vi "Final-MurphyE-Main.vi"() -> ()   [LabVIEW 2019]
uses:
  <vilib>/Analysis/1siggen.llb/Ramp Pattern by Samples.vi
  <vilib>/Utility/file.llb/Write Delimited Spreadsheet (DBL).vi
  <vilib>/Analysis/NI_AALBase.lvlib
panel:
  out "Inductor Value":string
  out "Capacitor Value":string
  out "Resistor  Value":string
  out "Results":cluster{"Ramp Pattern":dbl[], dbl[]}[](graph)
  out "parameter array":dbl[](array[numeric])
  out "standard output array":dbl[][](array[numeric])
  out "standard output":string
  out "command\nstring":string
  out "appended array":dbl[][](array[numeric])
  out "Multi1? 2":refnum<visa-resource-name>
  out "LogSpacedFreqList":dbl[](array[numeric])
  out "Multi1?":refnum<visa-resource-name>
  out "FG missing?":bool
  out "FG FOUND":bool
  out "Multimeter(s) Missing":bool
  out "2 Multimeters Found 2":bool
  out "Multimeters COM Port Array":refnum<visa-resource-name>[](array[refnum])
  # "Eddie Murphy's RLC Circuit Solver"
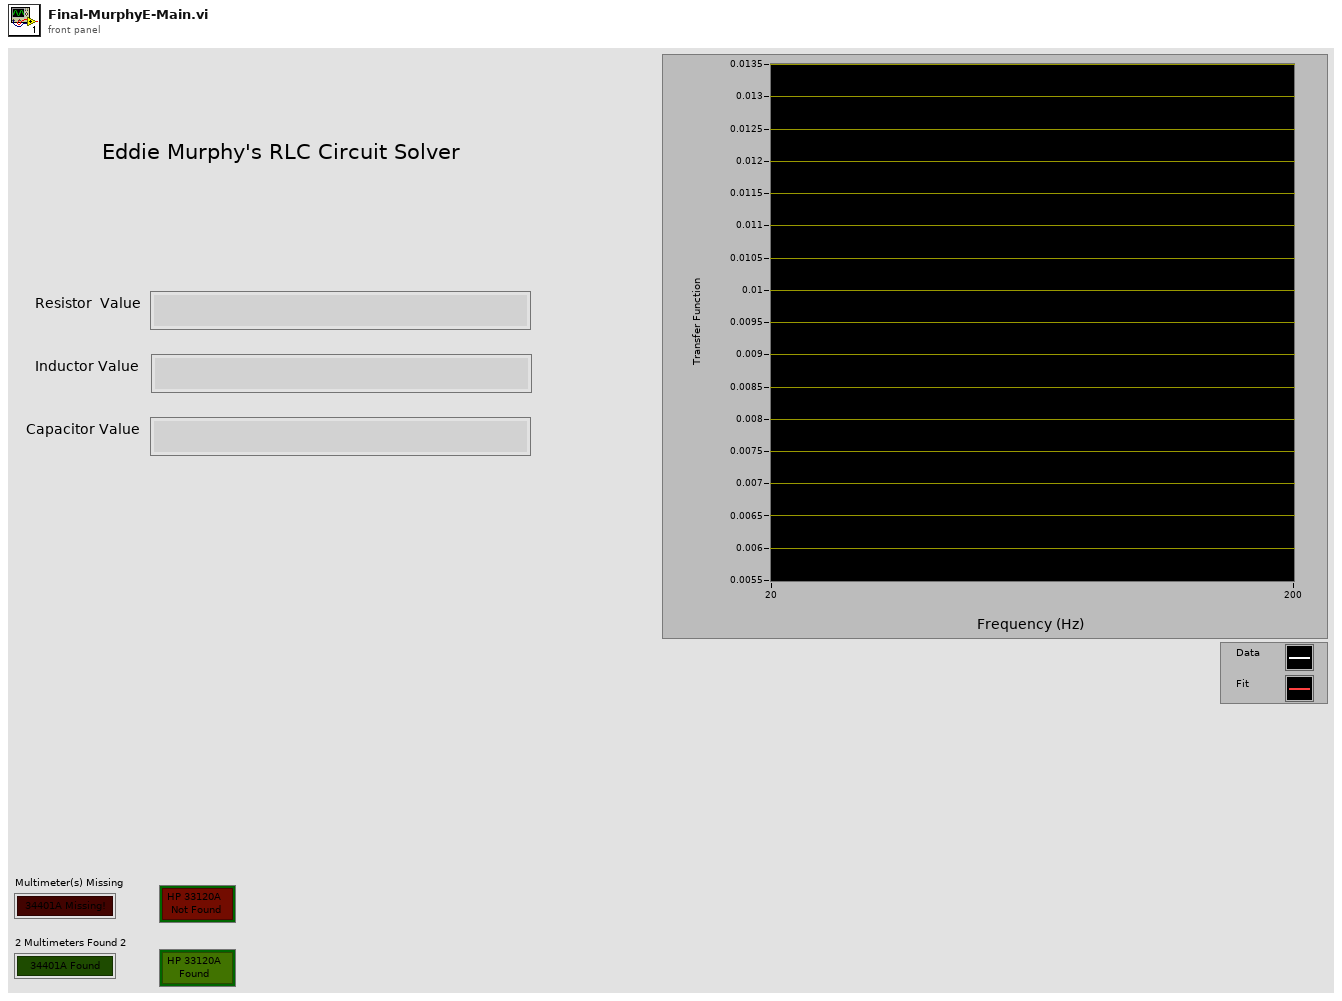
[diagram p1: front panel]
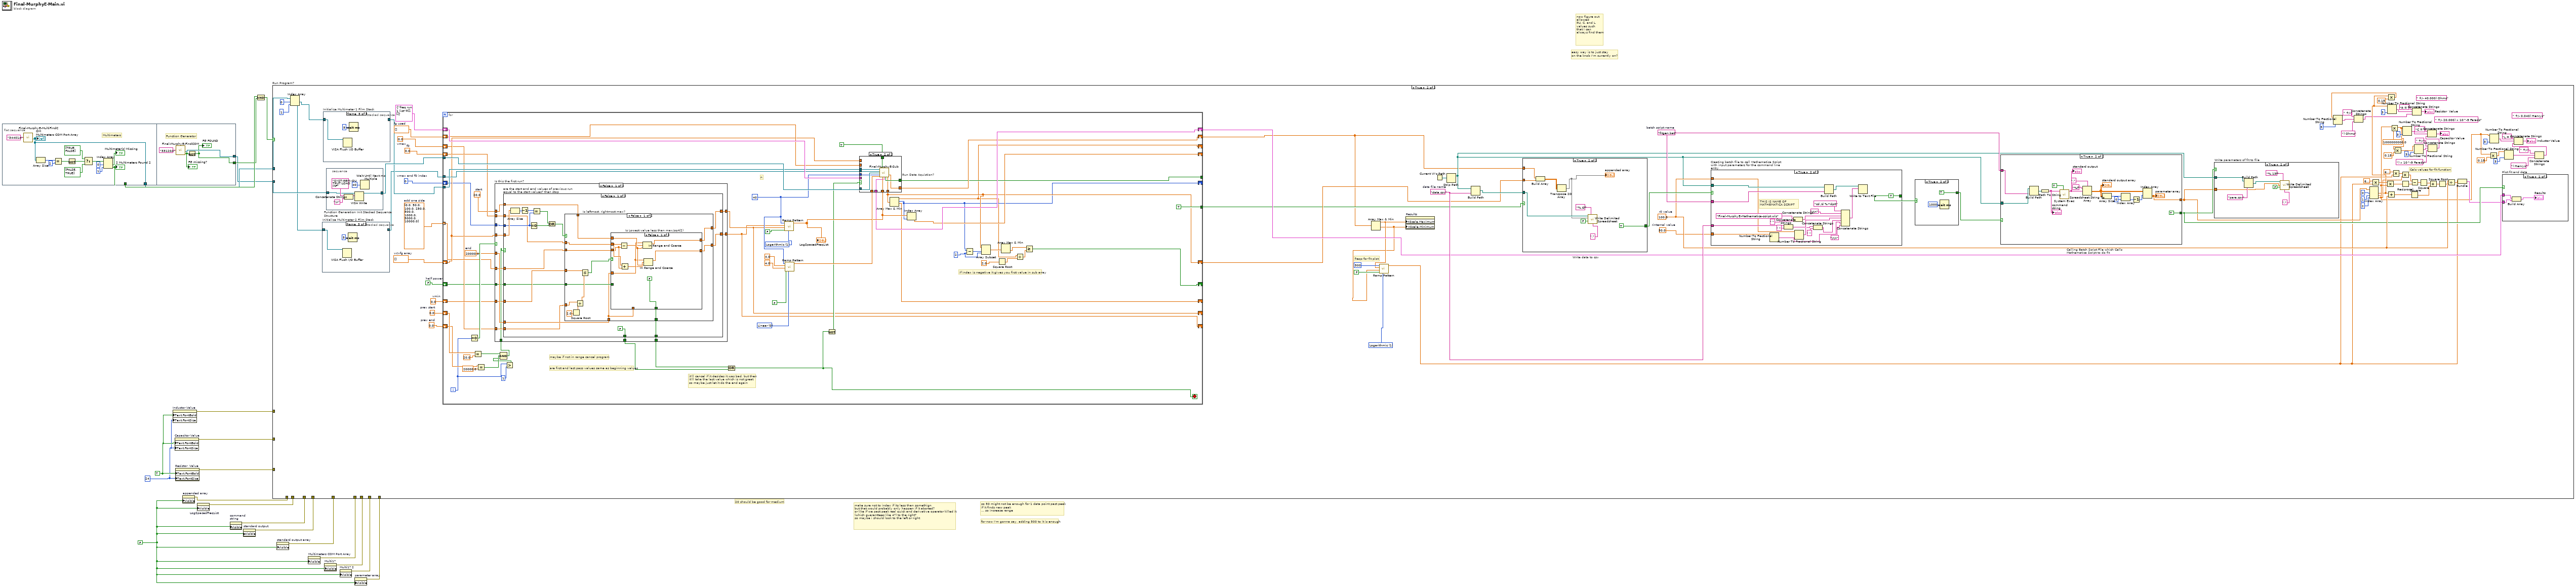
[diagram p0: block diagram]
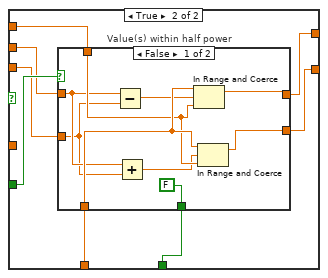
[diagram p3: hidden frame]
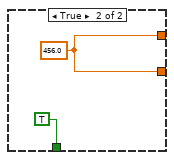
[diagram p4: hidden frame]
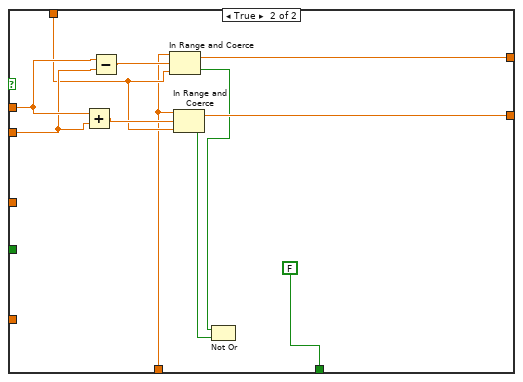
[diagram p5: hidden frame]
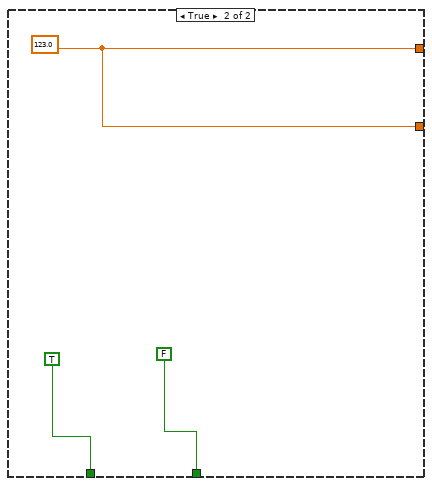
[diagram p6: hidden frame]
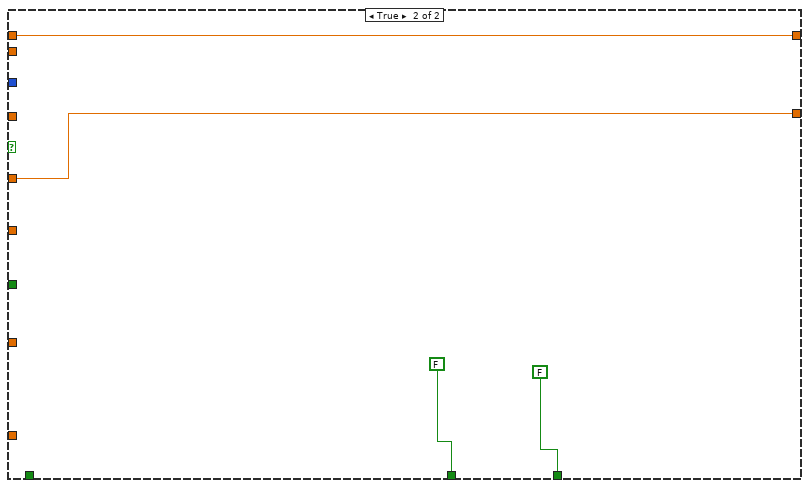
[diagram p7: hidden frame]
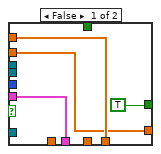
[diagram p8: hidden frame]
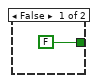
[diagram p11: hidden frame]
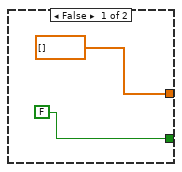
[diagram p12: hidden frame]
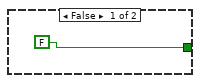
[diagram p13: hidden frame]
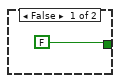
[diagram p14: hidden frame]
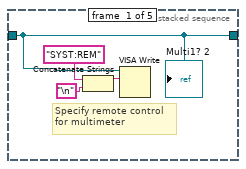
[diagram p15: hidden frame]
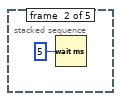
[diagram p16: hidden frame]
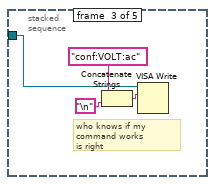
[diagram p17: hidden frame]
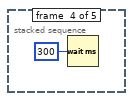
[diagram p18: hidden frame]
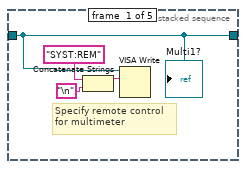
[diagram p19: hidden frame]
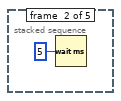
[diagram p20: hidden frame]
diagram:
  w3 = u32 24 ("Text.Font:Size")
  w4 = TRUE
  w7 = FALSE
  # "for now I'm gonna say, adding 500 to it is enough"
  # "so 50 might not be enough for 1 data point past peak\nif it finds new peak \n... so increase range"
  # "make sure not to index if its less than somethign\nbut that would probably only happen if it aborted?\nor like if we past peak real quick and derivative operator killed it (which guaranttees like 4?) to the right?\nso maybe i should look to the left or right"
  # "20 should be good for medium"
  # "easy way is to just stay \non the knob I'm currently on?"
  # "now figure out\nallowed\nRU, C, and L\nvalues such \nthat I can \nalways find them"
  n1 = flat-sequence {
    tunnel: [w22] -> w20
    tunnel: [w21] -> w18
    tunnel: [w36] -> w16
    tunnel: [w34] -> w19
    frame #0 {
      # "Multimeters"
      n2 = call "Final-MurphyE-MultiFindCOM.vi"("Name of Desired\nInstrument"="34401A" ("y")) -> ("Desired COM Port Array"=w21:refnum<visa-resource-name>[])  [unwired: 3 out]
      "Multimeters COM Port Array" <- w21
      n3 = Array Size(array=w21) -> (size(s)=w26:i32)
      n4 = Equal?(x=w26, y=2) -> (x = y?=w24:bool)
      n5 = Not(x=w24) -> (.not. x?=w23:bool)
      n6 = Select(t=bool[] [TRUE, FALSE], s=w23, f=bool[] [FALSE, TRUE]) -> (s? t:f=w30:bool[])
      n7 = Index Array(array=w30, index #1=0 ("index"), index #2=1) -> (element #1=→"Multimeter(s) Missing":bool, element #2=w22:bool)
      "2 Multimeters Found 2" <- w22
    }
    frame #1 {
      # "Function Generator"
      n8 = call "Final-MurphyE-FindCOM.vi"("Name of Desired\nInstrument"="33120A" ("y")) -> ("Desired \nCOM Port"=w36:refnum<visa-resource-name>, "Instrument\nNot Found"=w35:bool)  [unwired: 2 out]
      "FG missing?" <- w35
      n9 = Not(x=w35) -> (.not. x?=w34:bool)
      "FG FOUND" <- w34
    }
  }
  n10 = property on="Inductor Value" class="Str"("Text.FontBold"=w4, "Text.FontSize"=w3) -> (error out=w2:errorcluster)  [unwired: 2 in, 1 out]
  n11 = property on="Capacitor Value" class="Str"("Text.FontBold"=w4, "Text.FontSize"=w3) -> (error out=w1:errorcluster)  [unwired: 2 in, 1 out]
  n12 = property on="Resistor  Value" class="Str"("Text.FontBold"=w4, "Text.FontSize"=w3) -> (error out=w5:errorcluster)  [unwired: 2 in, 1 out]
  n13 = property on="appended array" class="Arr (strict)"("Visible"=w7) -> (error out=w14:errorcluster)  [unwired: 2 in, 1 out]
  n14 = property on="LogSpacedFreqList" class="Arr (strict)"("Visible"=w7) -> (error out=w15:errorcluster)  [unwired: 2 in, 1 out]
  n15 = property on="command\nstring" class="Str"("Visible"=w7) -> (error out=w13:errorcluster)  [unwired: 2 in, 1 out]
  n16 = property on="standard output" class="Str"("Visible"=w7) -> (error out=w12:errorcluster)  [unwired: 2 in, 1 out]
  n17 = Compound Arithmetic op=AND(w20, w19) -> (w17:bool)
  n18 = property on="standard output array" class="Arr (strict)"("Visible"=w7) -> (error out=w11:errorcluster)  [unwired: 2 in, 1 out]
  n19 = property on="Multimeters COM Port Array" class="Arr (strict)"("Visible"=w7) -> (error out=w8:errorcluster)  [unwired: 2 in, 1 out]
  n20 = property on="Multi1?" class="VISAName"("Visible"=w7) -> (error out=w10:errorcluster)  [unwired: 2 in, 1 out]
  n21 = property on="Multi1? 2" class="VISAName"("Visible"=w7) -> (error out=w9:errorcluster)  [unwired: 2 in, 1 out]
  n22 = property on="parameter array" class="Arr (strict)"("Visible"=w7) -> (error out=w6:errorcluster)  [unwired: 2 in, 1 out]
  n23 = case "Run Program?" shown="True" w17 {
    tunnel: w18 -> [_ w133]
    tunnel: w16 -> [_ w132]
    tunnel: w15 -> [_ _]
    tunnel: w14 -> [_ _]
    tunnel: w13 -> [_ _]
    tunnel: w12 -> [_ _]
    tunnel: w11 -> [_ _]
    tunnel: w10 -> [_ _]
    tunnel: w9 -> [_ _]
    tunnel: w8 -> [_ _]
    tunnel: w6 -> [_ _]
    tunnel: w5 -> [_ _]
    tunnel: w2 -> [_ _]
    tunnel: w1 -> [_ _]
    frame False {
    }
    frame True {
      w62 = FALSE  # half power
      w63 = 0.0  # prev end
      w64 = 0.0  # prev start
      w65 = 0.0  # vmin
      w66 = dbl[] [0.0, 50.0, 100.0, 250.0, 500.0, 1000.0, 5000.0, 10000.0]  # add one side
      w73 = u16 1 items=["Linear", "Logarithmic"] ("type")
      w80 = dbl[] []  # fg used
      w82 = 0.0  # vmax
      w83 = 0.0  # f0
      w84 = 0  # vmax and f0 index
      w85 = dbl[] []  # vr/vfg array
      w86 = 50.0  # rinternal value
      (unwired) " +/- 0.040) Henrys" ("string")
      (unwired) " +/- 20.000) x 10^-9 Farads" ("string")
      (unwired) " +/- 40.000) Ohms" ("string")
      w118 = 100.0  # r0 value
      w126 = "fitgen.bat"  # batch script name
      w123 = "data.csv"  # data file name
      # "freqs for fit plot"
      # "Calc values for fit function"
      n24 = Index Array(array=w133, index #1=0 ("index"), index #2=1 ("index")) -> (element #1=w131:refnum<visa-resource-name>, element #2=w130:refnum<visa-resource-name>)
      n25 = stacked-sequence "Initialize Multimeter 2 Film Stack" {
        tunnel: w130 -> [w362 _ w367 _ w372]
        tunnel: [w362 _ _ _ _] -> w75
        frame #0 {
          # "Specify remote control\nfor multimeter"
          n26 = Concatenate Strings("SYST:REM", "\n") -> (w365:string)
          n27 = VISA Write(VISA resource name=w362, write buffer=w365) -> ()  [unwired: 1 in, 3 out]
          "Multi1? 2" <- w362
        }
        frame #1 {
          n28 = Wait (ms)(milliseconds to wait=u32 5 ("millisecond multiple")) -> ()  [unwired: 1 out]
        }
        frame #2 {
          # "who knows if my command works\nis right"
          n29 = Concatenate Strings("conf:VOLT:ac", "\n") -> (w368:string)
          n30 = VISA Write(VISA resource name=w367, write buffer=w368) -> ()  [unwired: 1 in, 3 out]
        }
        frame #3 {
          n31 = Wait (ms)(milliseconds to wait=u32 300 ("millisecond multiple")) -> ()  [unwired: 1 out]
        }
        frame #4 {
          n32 = VISA Flush I/O Buffer(VISA resource name=w372) -> ()  [unwired: 2 in, 2 out]
          n33 = Wait (ms)(milliseconds to wait=u32 5 ("millisecond multiple")) -> ()  [unwired: 1 out]
        }
      }
      n34 = stacked-sequence "Initialize Multimeter 1 Film Stack" {
        tunnel: w131 -> [w380 _ w385 _ w390]
        tunnel: [w380 _ _ _ _] -> w76
        frame #0 {
          # "Specify remote control\nfor multimeter"
          n35 = Concatenate Strings("SYST:REM", "\n") -> (w383:string)
          n36 = VISA Write(VISA resource name=w380, write buffer=w383) -> ()  [unwired: 1 in, 3 out]
          "Multi1?" <- w380
        }
        frame #1 {
          n37 = Wait (ms)(milliseconds to wait=u32 5 ("millisecond multiple")) -> ()  [unwired: 1 out]
        }
        frame #2 {
          # "who knows if my command works\nis right"
          n38 = Concatenate Strings("conf:VOLT:ac", "\n") -> (w386:string)
          n39 = VISA Write(VISA resource name=w385, write buffer=w386) -> ()  [unwired: 1 in, 3 out]
        }
        frame #3 {
          n40 = Wait (ms)(milliseconds to wait=u32 300 ("millisecond multiple")) -> ()  [unwired: 1 out]
        }
        frame #4 {
          n41 = VISA Flush I/O Buffer(VISA resource name=w390) -> ()  [unwired: 2 in, 2 out]
          n42 = Wait (ms)(milliseconds to wait=u32 5 ("millisecond multiple")) -> ()  [unwired: 1 out]
        }
      }
      n43 = stacked-sequence "Function Generation Init Stacked Sequence Structure" {
        tunnel: w132 -> [w376]
        tunnel: [w374] -> w77
        frame #0 {
          n44 = Concatenate Strings("SYST:REM;:OUTPUT:LOAD INF", "\n") -> (w378:string)
          n45 = VISA Write(VISA resource name=w376, write buffer=w378) -> (VISA resource name out=w374:refnum<visa-resource-name>)  [unwired: 1 in, 2 out]
          n46 = Wait Until Next ms Multiple(millisecond multiple=u32 40) -> ()  [unwired: 1 out]
        }
      }
      n47 = for {
        tunnel: [w181] -> _
        shift-right: [w150] -> w78
        shift-left: w85 -> [w172]
        shift-right: [w148] -> _
        shift-left: w84 -> [w171]
        shift-right: [w175] -> _
        shift-left: w83 -> [w173]
        shift-right: [w141] -> _
        shift-left: w82 -> [w164]
        shift-right: [w185] -> w79
        shift-left: cluster{"freq run 1 list":dbl[], dbl[]} {"freq run 1 list"=[], []} ("vr/vfg rms Cluster for graph") -> [w184]
        shift-right: [w183] -> w68
        shift-left: w80 -> [w182]
        tunnel: w77 -> [w179]
        tunnel: w76 -> [w178]
        tunnel: w75 -> [w177]
        tunnel: [TRUE] -> w74
        tunnel: w66 -> [w168] mode=indexing
        shift-right: [w167] -> _
        shift-left: w65 -> [w166]
        shift-right: [w160] -> _
        shift-left: w64 -> [w158]
        shift-right: [w159] -> _
        shift-left: w63 -> [w156]
        shift-right: [w140] -> _
        shift-left: w62 -> [w139]
        i -> [w138]
        stop <- w161 stop-if-true
        w147 = 2
        w165 = 40
        w169 = 20000.0  # end
        w170 = 20.0  # start
        w187 = u16 1 items=["Linear", "Logarithmic"] ("type")
        w192 = u16 0 items=["Linear", "Logarithmic"] ("type")
        # "if index is negative it gives you first value in sub array"
        # "are first and last pass values same as beginning values"
        # "it'll cancel if it desides it was bad, but then \nit'll take the last value which is not great \nso maybe just let it do the end again"
        # "maybe if not in range cancel program"
        # "n"
        n48 = Equal To 0?(x=w138) -> (x = 0?=w174:bool)
        n49 = Equal?(x=w158, y=20.0) -> (x = y?=w154:bool)
        n50 = Equal?(x=w156, y=20000.0) -> (x = y?=w153:bool)
        n51 = Greater?(x=w138, y=1) -> (0:w136:bool)
        n52 = Compound Arithmetic op=AND(w154, w153, w136) -> (w152:bool)
        n53 = case "Is this the first run?" shown="False" w174 {
          tunnel: [w201 w285] -> w160
          tunnel: [w200 w284] -> w159
          tunnel: w173 -> [w205 _]
          tunnel: w172 -> [w207 _]
          tunnel: w171 -> [w206 _]
          tunnel: w170 -> [w204 w285]
          tunnel: w169 -> [w203 w284]
          tunnel: w168 -> [w202 _]
          tunnel: w166 -> [w199 _]
          tunnel: w164 -> [w198 _]
          tunnel: [w197 FALSE] -> w163
          tunnel: w152 -> [w196 _]
          tunnel: [w195 FALSE] -> w151
          tunnel: w139 -> [w194 _]
          frame False {
            n54 = case "are the start and end values of previous run equal to the start values? then stop" shown="False" w196 {
              tunnel: w207 -> [w224 _]
              tunnel: w206 -> [w221 _]
              tunnel: w205 -> [w218 _]
              tunnel: w204 -> [w217 _]
              tunnel: w203 -> [w216 _]
              tunnel: w202 -> [w215 _]
              tunnel: [w214 w281] -> w201
              tunnel: [w213 w281] -> w200
              tunnel: w199 -> [w212 _]
              tunnel: w198 -> [w211 _]
              tunnel: [w210 FALSE] -> w197
              tunnel: [FALSE TRUE] -> w195
              tunnel: w194 -> [w208 _]
              frame False {
                n55 = Array Size(array=w224) -> (size(s)=w223:i32)
                n56 = Decrement(x=w223) -> (x-1=w222:i32)
                n57 = Equal To 0?(x=w221) -> (x = 0?=w225:bool)
                n58 = Equal?(x=w222, y=w221) -> (x = y?=w220:bool)
                n59 = Or(x=w220, y=w225) -> (x .or. y?=w219:bool)
                n60 = case "Is leftmost, rightmost max?" shown="False" w219 {
                  tunnel: w218 -> [w229 w276]
                  tunnel: w217 -> [w230 w271]
                  tunnel: w216 -> [w226 w270]
                  tunnel: [w232 w278] -> w214
                  tunnel: [w231 w277] -> w213
                  tunnel: w215 -> [w228 w275]
                  tunnel: w212 -> [w239 _]
                  tunnel: w211 -> [w237 _]
                  tunnel: [w233 FALSE] -> w210
                  tunnel: w208 -> [w227 _]
                  frame False {
                    n61 = Square Root(x=2.0) -> (sqrt(x)=w235:dbl)
                    n62 = Divide(x=w237, y=w235) -> (x/y=w236:dbl)
                    n63 = Less Or Equal?(x=w239, y=w236) -> (x <= y?=w238:bool)
                    n64 = case "Is Lowest value less than max/sqrt(2)" shown="False" w238 {
                      tunnel: [FALSE w255] -> w233
                      tunnel: [w247 w254] -> w232
                      tunnel: [w246 w253] -> w231
                      tunnel: w226 -> [w244 _]
                      tunnel: w230 -> [w245 w251]
                      tunnel: w229 -> [w241 w250]
                      tunnel: w228 -> [w240 w249]
                      tunnel: w227 -> [_ w256]
                      tunnel: w226 -> [_ w252]
                      frame False {
                        n65 = Subtract(x=w241, y=w240) -> (x-y=w243:dbl)
                        n66 = Add(x=w241, y=w240) -> (x+y=w242:dbl)
                        n67 = In Range and Coerce(upper limit=w244, x=w243, lower limit=w245) -> (coerced(x)=w247:dbl)  [unwired: 1 out]
                        n68 = In Range and Coerce(upper limit=w244, x=w242, lower limit=w245) -> (coerced(x)=w246:dbl)  [unwired: 1 out]
                      }
                      frame True {
                        n69 = case "Value(s) within half power" shown="False" w256 {
                          tunnel: [FALSE TRUE] -> w255
                          tunnel: [w259 w266] -> w254
                          tunnel: [w260 w266] -> w253
                          tunnel: w252 -> [w264 _]
                          tunnel: w251 -> [w263 _]
                          tunnel: w250 -> [w258 _]
                          tunnel: w249 -> [w257 _]
                          frame False {
                            n70 = Subtract(x=w258, y=w257) -> (x-y=w262:dbl)
                            n71 = Add(x=w258, y=w257) -> (x+y=w261:dbl)
                            n72 = In Range and Coerce(upper limit=w264, x=w262, lower limit=w263) -> (coerced(x)=w259:dbl)  [unwired: 1 out]
                            n73 = In Range and Coerce(upper limit=w264, x=w261, lower limit=w263) -> (coerced(x)=w260:dbl)  [unwired: 1 out]
                          }
                          frame True {
                            w266 = 456.0
                          }
                        }
                      }
                    }
                  }
                  frame True {
                    n74 = Add(x=w276, y=w275) -> (x+y=w274:dbl)
                    n75 = Subtract(x=w276, y=w275) -> (x-y=w273:dbl)
                    n76 = In Range and Coerce(upper limit=w270, x=w273, lower limit=w271) -> (coerced(x)=w278:dbl, In Range?=w268:bool)
                    n77 = In Range and Coerce(upper limit=w270, x=w274, lower limit=w271) -> (coerced(x)=w277:dbl, In Range?=w269:bool)
                    n78 = Not Or(1:w269, 2:w268) -> ()  [unwired: 1 out]
                  }
                }
              }
              frame True {
                w281 = 123.0
              }
            }
          }
          frame True {
          }
        }
        n79 = Compound Arithmetic op=OR(w163, w151) -> (w161:bool)
        n80 = call-poly <vilib>:"Ramp Pattern.vi"("type"=w187, "exclude end?"=FALSE, "start"=w160, "end"=w159, "samples"=w165) -> ("Ramp Pattern"=w186:dbl[])  [unwired: 5 in, 1 out]
        "LogSpacedFreqList" <- w186
        n81 = call-poly <vilib>:"Ramp Pattern.vi"("type"=w192, "exclude end?"=FALSE, "start"=4.0, "end"=4.0, "samples"=w165) -> ("Ramp Pattern"=w188:dbl[])  [unwired: 5 in, 1 out]
        n82 = Not(x=w161) -> (.not. x?=w162:bool)
        n83 = case "Run Data Aquistion?" shown="True" w162 {
          tunnel: w178 -> [_ w300]
          tunnel: w177 -> [_ w299]
          tunnel: w179 -> [_ w298]
          tunnel: w188 -> [_ w297]
          tunnel: TRUE ("Measure? 2 Init Value") -> [_ w296]
          tunnel: [TRUE w295] -> w181
          tunnel: w165 -> [_ w294]
          tunnel: w186 -> [_ w293]
          tunnel: [w289 w292] -> w150
          tunnel: w172 -> [w289 _]
          tunnel: [w287 w291] -> w185
          tunnel: w184 -> [w287 _]
          tunnel: [w286 w290] -> w183
          tunnel: w182 -> [w286 _]
          frame False {
          }
          frame True {
            n84 = call "Final-MurphyE-Sub.vi"("multimeter 1 in"=w300, "Measure? 2 Init Value"=w296, "multimeter 2 in"=w299, "function gen in"=w298, "n"=w294, "vp-pk to pk array of values"=w297, "freq array input"=w293) -> ("freq array output (used)"=w290:dbl[], "vr/vfg rms Cluster for graph"=w291:cluster{"freq run 1 list":dbl[], dbl[]}, "Run 2 True Condition Measure Button"=w295:bool, "vr/vfg array"=w292:dbl[])  [unwired: 1 in, 4 out]
          }
        }
        n85 = Array Max & Min(array=w150) -> (max value=w141:dbl, max index (indices)=w148:i32, min value=w167:dbl)  [unwired: 1 out]
        n86 = Index Array(array=w186, index=w148) -> (element=w175:dbl)
        n87 = Subtract(x=w148, y=w147) -> (x-y=w149:i32)
        n88 = Array Subset(array=w150, index=w149, length=w147) -> (w146:dbl[])
        n89 = Square Root(x=2.0) -> (sqrt(x)=w143:dbl)
        n90 = Array Max & Min(array=w146) -> (min value=w145:dbl)  [unwired: 3 out]
        n91 = Divide(x=w141, y=w143) -> (x/y=w144:dbl)
        n92 = Greater Or Equal?(x=w145, y=w144) -> (x >= y?=w140:bool)
      }
      n93 = Array Max & Min(array=w68) -> (max value=w70:dbl, min value=w69:dbl)  [unwired: 2 out]
      n94 = call-poly <vilib>:"Ramp Pattern.vi"("type"=w73, "exclude end?"=FALSE, "start"=w69, "end"=w70, "samples"=500) -> ("Ramp Pattern"=w67:dbl[])  [unwired: 5 in, 1 out]
      n95 = property on="Results" class="XYGraph (strict)"("XScale.Maximum"=w70, "XScale.Minimum"=w69) -> ()  [unwired: 2 in, 2 out]
      n96 = Current VI's Path() -> (path=w128:path)
      n97 = Strip Path(path=w128) -> (stripped path=w104:path)  [unwired: 1 out]
      n98 = Build Path(base path=w104, name or relative path=w123) -> (appended path=w127:path)
      n99 = case "Write data to csv" shown="True" w74 {
        tunnel: w68 -> [_ w361]
        tunnel: w78 -> [_ w360]
        tunnel: [FALSE TRUE] -> w129
        tunnel: w127 -> [_ w356]
        frame False {
        }
        frame True {
          n100 = Build Array(w361, w360) -> (w355:dbl[][])
          n101 = Transpose 2D Array(2D array=w355) -> (transposed array=w354:dbl[][])
          "appended array" <- w354
          n102 = call-poly <vilib>:"Write Delimited Spreadsheet.vi"("file path (dialog if empty)"=w356, "format (%.3f)"="%.6f", "2D data"=w354, "append to file? (new file:F)"=FALSE, "delimiter (\\t)"="," ("delimiter (\\t)")) -> ()  [unwired: 9 in, 2 out]
        }
      }
      n103 = case "Creating batch file to call Mathematica Script with input parameters for the command line entry" shown="True" w129 {
        tunnel: [FALSE TRUE] -> w125
        tunnel: w104 -> [_ w346]
        tunnel: w126 -> [_ w345]
        tunnel: w123 -> [_ w344]
        tunnel: w118 -> [_ w341]
        tunnel: w86 -> [_ w332]
        frame False {
        }
        frame True {
          # "THIS IS NAME OF \nMATHEMATICA SCRIPT"
          n104 = Number To Fractional String(number=w332) -> (F-format string=w339:string)  [unwired: 3 in]
          n105 = Concatenate Strings(w344, " " ("string")) -> (w342:string)
          n106 = Concatenate Strings("Final-MurphyE-Mathematica-script.wls" ("string"), " " ("string")) -> (w337:string)
          n107 = Number To Fractional String(number=w341) -> (F-format string=w335:string)  [unwired: 3 in]
          n108 = Concatenate Strings(w335, " " ("string")) -> (w334:string)
          n109 = Build Path(base path=w346, name or relative path=w345) -> (appended path=w350:path)
          n110 = Concatenate Strings("cd /d %~dp0" ("string"), "\r\n", w337, w342, w334, w339, "\r\n") -> (w349:string)
          n111 = Write to Text File(file (use dialog)=w350, text=w349) -> ()  [unwired: 2 in, 3 out]
        }
      }
      n112 = case shown="True" w125 {
        tunnel: [FALSE TRUE] -> w124
        frame False {
        }
        frame True {
          n113 = Wait (ms)(milliseconds to wait=u32 1000) -> ()  [unwired: 1 out]
        }
      }
      n114 = case "Calling Batch Script File which Calls Mathematica Script to do fit" shown="True" w124 {
        tunnel: w104 -> [_ w319]
        tunnel: w126 -> [_ w318]
        tunnel: [FALSE TRUE] -> w103
        tunnel: [dbl[] [] w316] -> w101
        frame False {
        }
        frame True {
          n115 = Build Path(base path=w319, name or relative path=w318) -> (appended path=w330:path)
          n116 = Path To String(path=w330) -> (string=w328:string)
          "command\nstring" <- w328
          n117 = call <vilib>:"System Exec.vi"("wait until completion? (T)"=TRUE, "command line"=w328) -> ("standard output"=w327:string)  [unwired: 6 in, 3 out]
          "standard output" <- w327
          n118 = Spreadsheet String To Array(delimiter (Tab)=",", format string="%f", spreadsheet string=w327) -> (array=w321:dbl[][])  [unwired: 1 in]
          "standard output array" <- w321
          n119 = Array Size(array=w321) -> (size(s)=w324:i32[])
          n120 = Index Array(array=w324, index=0) -> (element=w322:i32)
          n121 = Decrement(x=w322) -> (x-1=w320:i32)
          n122 = Index Array(array=w321, index (row)=w320) -> (element=w316:dbl[])  [unwired: 1 in]
          "parameter array" <- w316
        }
      }
      n123 = case "Write parameters of fit to file" shown="True" w103 {
        tunnel: w104 -> [_ w303]
        tunnel: w101 -> [_ w302]
        frame False {
        }
        frame True {
          n124 = Build Path(base path=w303, name or relative path="para.csv") -> (appended path=w305:path)
          n125 = call-poly <vilib>:"Write Delimited Spreadsheet.vi"("file path (dialog if empty)"=w305, "format (%.3f)"="%.13f", "1D data"=w302, "append to file? (new file:F)"=FALSE, "delimiter (\\t)"="," ("delimiter (\\t)")) -> ()  [unwired: 9 in, 2 out]
        }
      }
      n126 = Index Array(array=w101, index #1=0 ("index"), index #2=1 ("index"), index #3=2 ("index")) -> (element #1=w61:dbl, element #2=w94:dbl, element #3=w45:dbl)
      n127 = Multiply(x=6.283185307179586, y=w67) -> (x*y=w107:dbl[])
      n128 = Multiply(x=w107, y=w94) -> (x*y=w106:dbl[])
      n129 = Multiply(x=w61, y=0.15) -> (x*y=w58:dbl)
      n130 = Number To Fractional String(number=w58, precision (6)=i16 3) -> (F-format string=w57:string)  [unwired: 2 in]
      n131 = Concatenate Strings(" +/-" ("element"), w57, ") Ohms" ("element")) -> (w54:string)
      n132 = Add(x=w61, y=w118) -> (x+y=w117:dbl)
      n133 = Number To Fractional String(number=w61, precision (6)=i16 3) -> (F-format string=w100:string)  [unwired: 2 in]
      n134 = Multiply(x=w94, y=1000000000.0) -> (x*y=w53:dbl)
      n135 = Multiply(x=6.283185307179586, y=w67) -> (x*y=w113:dbl[])
      n136 = Multiply(x=w53, y=0.15) -> (x*y=w51:dbl)
      n137 = Multiply(x=w113, y=w45) -> (x*y=w112:dbl[])
      n138 = Reciprocal(x=w106) -> (1/x=w109:dbl[])
      n139 = Number To Fractional String(number=w53, precision (6)=i16 3) -> (F-format string=w97:string)  [unwired: 2 in]
      n140 = Square(x=w117) -> (x^2=w115:dbl)
      n141 = Subtract(x=w112, y=w109) -> (x-y=w111:dbl[])
      n142 = Concatenate Strings("R = (" ("string"), w100, w54) -> (→"Resistor  Value":string)
      n143 = Number To Fractional String(number=w51, precision (6)=i16 3) -> (F-format string=w49:string)  [unwired: 2 in]
      n144 = Square(x=w111) -> (x^2=w110:dbl[])
      n145 = Concatenate Strings(" +/-" ("element"), w49, ") x 10^-9 Farads" ("element")) -> (w46:string)
      n146 = Concatenate Strings("C = (" ("string"), w97, w46) -> (→"Capacitor Value":string)
      n147 = Add(x=w110, y=w115) -> (x+y=w116:dbl[])
      n148 = Square Root(x=w116) -> (sqrt(x)=w119:dbl[])
      n149 = Divide(x=w118, y=w119) -> (x/y=w105:dbl[])
      n150 = Bundle("Ramp Pattern"=w67, w105) -> (w102:cluster{"Ramp Pattern":dbl[], dbl[]})  [unwired: 1 in]
      n151 = Multiply(x=w45, y=0.15) -> (x*y=w43:dbl)
      n152 = Number To Fractional String(number=w45, precision (6)=i16 3) -> (F-format string=w92:string)  [unwired: 2 in]
      n153 = case "Plot fit and data" shown="True" w103 {
        tunnel: w79 -> [_ w309]
        tunnel: w102 -> [_ w308]
        frame False {
        }
        frame True {
          n154 = Build Array(w309, w308) -> (→"Results":cluster{"Ramp Pattern":dbl[], dbl[]}[])
        }
      }
      n155 = Number To Fractional String(number=w43, precision (6)=i16 3) -> (F-format string=w41:string)  [unwired: 2 in]
      n156 = Concatenate Strings(" +/-" ("element"), w41, ") Henrys" ("element")) -> (w38:string)
      n157 = Concatenate Strings("L = (" ("string"), w92, w38) -> (→"Inductor Value":string)
    }
  }
